vi "AR-DO-close.vi"(8 "error in (no error)":errorcluster, 11 "DO task in":refnum<k21>) -> (0 "error out":errorcluster)   [LabVIEW 2021]
uses:
  <resource>/objmgr/daqmx.rc
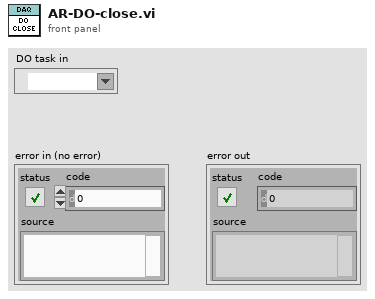
[diagram p1: front panel]
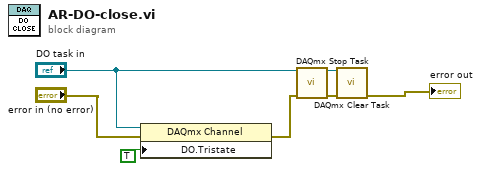
[diagram p0: block diagram]
diagram:
  n1 = property class="DAQmx Channel"(reference="DO task in", error in="error in (no error)", "DO.Tristate"=TRUE) -> (error out=w7:errorcluster)  [unwired: 1 out]
  n2 = call <vilib>:"DAQmx Stop Task.vi"("task/channels in"="DO task in", "error in"=w7) -> ("task out"=w3:refnum<k21>, "error out"=w4:errorcluster)  [unwired: 12 in]
  n3 = call <vilib>:"DAQmx Clear Task.vi"("task in"=w3, "error in"=w4) -> ("error out"=→"error out":errorcluster)  [unwired: 13 in]
